vi "Meter-FunctionalTest.vi"(8 "error in (no error)":errorcluster, 11 "Meter-Test in":refnum<class "Meter-Test.lvclass">) -> (0 "error out":errorcluster, 3 "Meter-Test out":refnum<class "Meter-Test.lvclass">)   [LabVIEW 2013, in "Meter-Test.lvclass"]
uses:
  Meter-Test.lvclass
  Meter-Test.lvclass/Meter-Test.ctl
  Desktop/Meter test with feedack.llb/MGI Wait (U32).vi
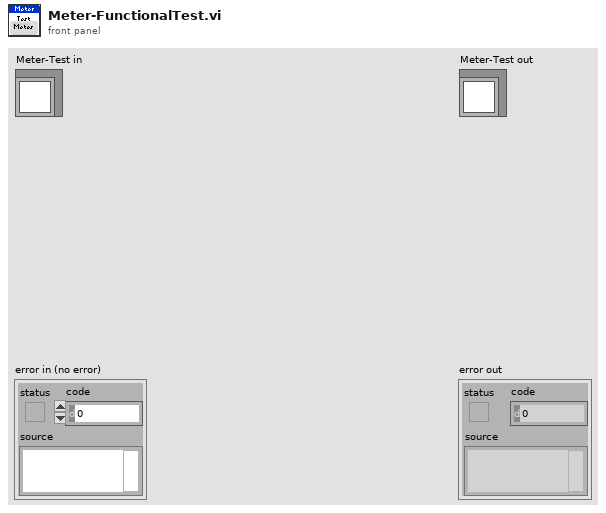
[diagram p1: front panel]
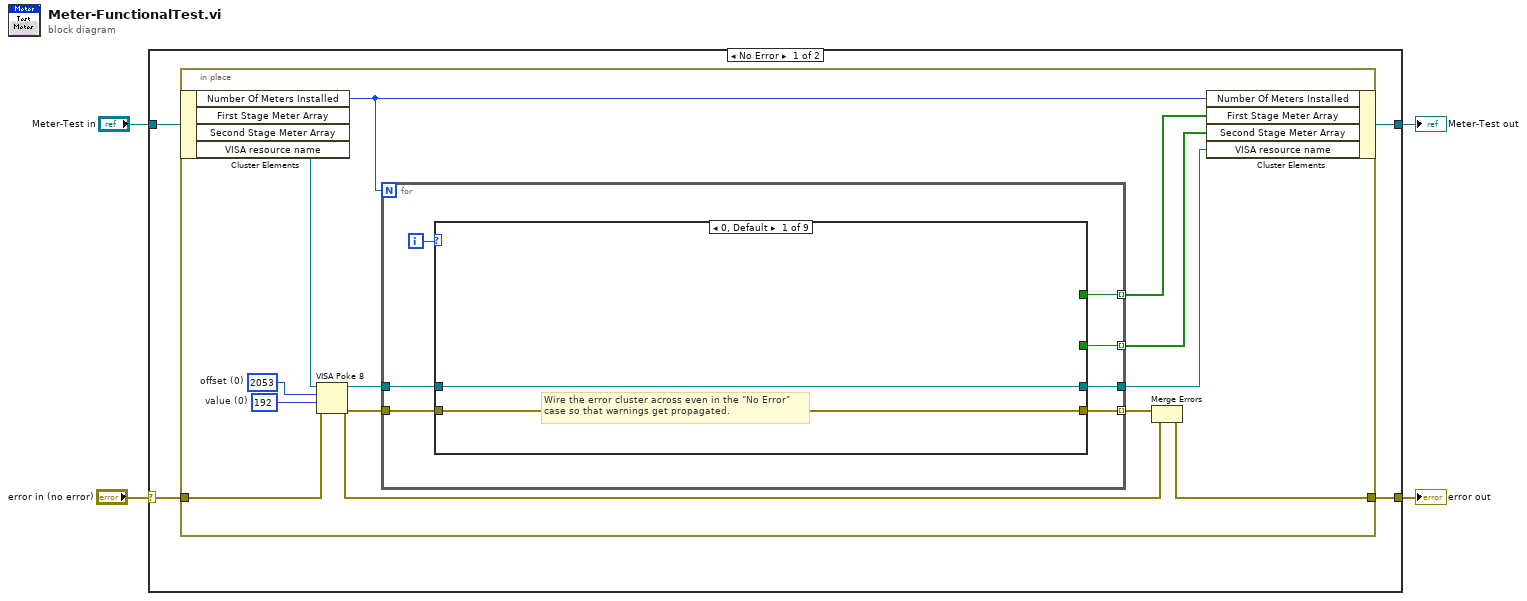
[diagram p0: block diagram]
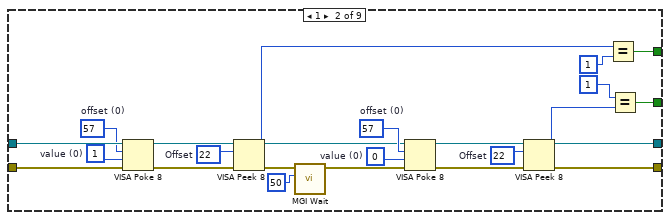
[diagram p2: hidden frame]
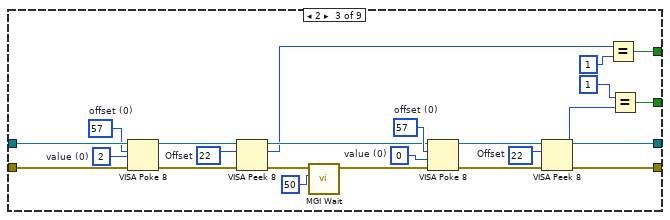
[diagram p3: hidden frame]
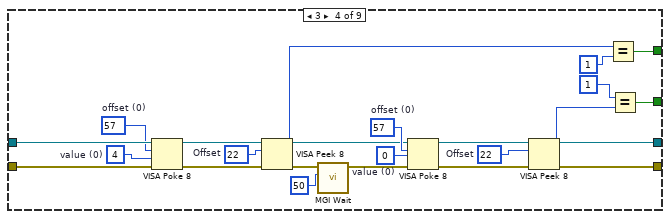
[diagram p4: hidden frame]
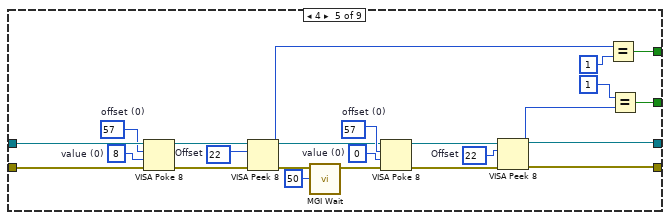
[diagram p5: hidden frame]
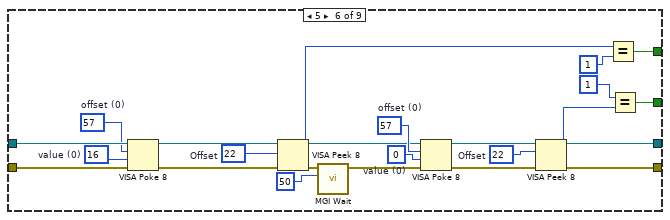
[diagram p6: hidden frame]
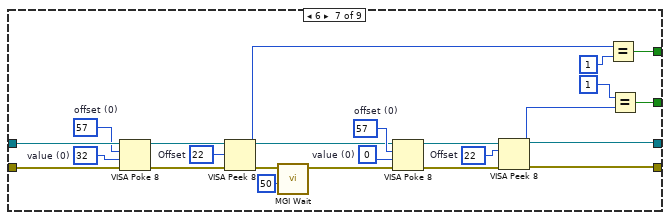
[diagram p7: hidden frame]
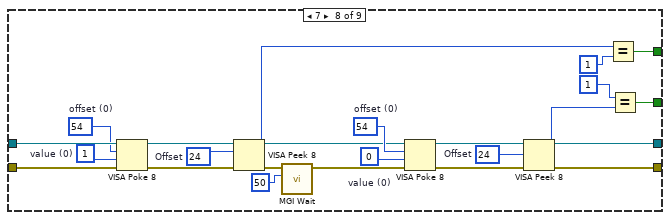
[diagram p8: hidden frame]
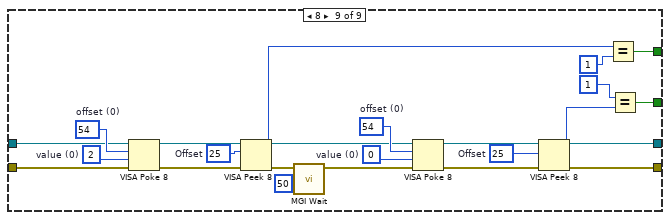
[diagram p9: hidden frame]
diagram:
  n1 = case shown="No Error" "error in (no error)" {
    selector: "error in (no error)" -> [w7 w222]
    tunnel: [w5 w222] -> w3
    tunnel: [w6 w221] -> w1
    tunnel: "Meter-Test in" -> [w8 w221]
    frame No Error {
      n2 = in-place {
        in-place-border: w7 -> [w15]
        in-place-border: [w11] -> w5
        w18 = u8 192  # value (0)
        w17 = u32 2053  # offset (0)
        # "Wire the error cluster across even in the \"No Error\"\ncase so that warnings get propagated."
        n3 = in-place-cluster #1(w8) -> ("Number Of Meters Installed"=w14:i32, "VISA resource name"=w13:refnum<visa-resource-name>)  [unwired: 2 out]
        n4 = VISA Poke 8(8:w15, 9:w18, 10:w17, 11:w13) -> (0:w20:errorcluster, 3:w16:refnum<visa-resource-name>)
        n5 = for {
          N: w14 -> [_]
          tunnel: [w27] -> w19 mode=indexing
          tunnel: w20 -> [w26]
          tunnel: w16 -> [w25]
          tunnel: [w23] -> w9 mode=indexing
          tunnel: [w22] -> w10 mode=indexing
          tunnel: [w21] -> w12
          i -> [w24]
          n6 = case shown="0, Default" w24 {
            tunnel: [w29 w52 w64 w88 w108 w132 w161 w180 w205] -> w27
            tunnel: w26 -> [w29 w51 w76 w100 w124 w148 w172 w196 w220]
            tunnel: w25 -> [w28 w50 w75 w99 w123 w147 w171 w195 w197]
            tunnel: [_ w33 w56 w80 w105 w129 w153 w177 w202] -> w23
            tunnel: [_ w30 w55 w81 w104 w128 w152 w176 w201] -> w22
            tunnel: [w28 w36 w59 w78 w101 w126 w150 w175 w200] -> w21
            frame 0, Default {
            }
            frame 1 {
              w39 = u32 22  # Offset
              w43 = u32 22  # Offset
              w45 = u8 0  # value (0)
              w46 = u32 57  # offset (0)
              w49 = u8 1  # value (0)
              w48 = u32 57  # offset (0)
              n7 = VISA Poke 8(8:w51, 9:w49, 10:w48, 11:w50) -> (0:w42:errorcluster, 3:w40:refnum<visa-resource-name>)
              n8 = VISA Peek 8(8:w42, 10:w43, 11:w40) -> (0:w41:errorcluster, 2:w31:u8, 3:w37:refnum<visa-resource-name>)
              n9 = call-poly "MGI Wait.vi"("ms"=u32 50, "Error In"=w41) -> ("Error Out"=w47:errorcluster)  [unwired: 5 in]
              n10 = VISA Poke 8(8:w47, 9:w45, 10:w46, 11:w37) -> (0:w52:errorcluster, 3:w38:refnum<visa-resource-name>)
              n11 = VISA Peek 8(10:w39, 11:w38) -> (2:w32:u8, 3:w36:refnum<visa-resource-name>)  [unwired: 1 in, 1 out]
              n12 = Equal?(x=w31, y=u8 1) -> (x = y?=w30:bool)
              n13 = Equal?(x=u8 1 ("y"), y=w32) -> (x = y?=w33:bool)
            }
            frame 2 {
              w67 = u32 22  # Offset
              w68 = u32 22  # Offset
              w70 = u8 0  # value (0)
              w71 = u32 57  # offset (0)
              w74 = u8 2  # value (0)
              w73 = u32 57  # offset (0)
              n14 = VISA Poke 8(8:w76, 9:w74, 10:w73, 11:w75) -> (0:w63:errorcluster, 3:w61:refnum<visa-resource-name>)
              n15 = VISA Peek 8(8:w63, 10:w68, 11:w61) -> (0:w62:errorcluster, 2:w54:u8, 3:w60:refnum<visa-resource-name>)
              n16 = call-poly "MGI Wait.vi"("ms"=u32 50, "Error In"=w62) -> ("Error Out"=w72:errorcluster)  [unwired: 5 in]
              n17 = VISA Poke 8(8:w72, 9:w70, 10:w71, 11:w60) -> (0:w66:errorcluster, 3:w65:refnum<visa-resource-name>)
              n18 = VISA Peek 8(8:w66, 10:w67, 11:w65) -> (0:w64:errorcluster, 2:w53:u8, 3:w59:refnum<visa-resource-name>)
              n19 = Equal?(x=w54, y=u8 1) -> (x = y?=w55:bool)
              n20 = Equal?(x=u8 1 ("y"), y=w53) -> (x = y?=w56:bool)
            }
            frame 3 {
              w92 = u32 22  # Offset
              w93 = u32 22  # Offset
              w95 = u8 0  # value (0)
              w87 = u32 57  # offset (0)
              w98 = u8 4  # value (0)
              w97 = u32 57  # offset (0)
              n21 = VISA Poke 8(8:w100, 9:w98, 10:w97, 11:w99) -> (0:w91:errorcluster, 3:w85:refnum<visa-resource-name>)
              n22 = VISA Peek 8(8:w91, 10:w93, 11:w85) -> (0:w90:errorcluster, 2:w77:u8, 3:w84:refnum<visa-resource-name>)
              n23 = call-poly "MGI Wait.vi"("ms"=u32 50, "Error In"=w90) -> ("Error Out"=w96:errorcluster)  [unwired: 5 in]
              n24 = VISA Poke 8(8:w96, 9:w95, 10:w87, 11:w84) -> (0:w89:errorcluster, 3:w86:refnum<visa-resource-name>)
              n25 = VISA Peek 8(8:w89, 10:w92, 11:w86) -> (0:w88:errorcluster, 2:w79:u8, 3:w78:refnum<visa-resource-name>)
              n26 = Equal?(x=w77, y=u8 1) -> (x = y?=w81:bool)
              n27 = Equal?(x=u8 1 ("y"), y=w79) -> (x = y?=w80:bool)
            }
            frame 4 {
              w115 = u32 22  # Offset
              w116 = u32 22  # Offset
              w118 = u8 0  # value (0)
              w119 = u32 57  # offset (0)
              w122 = u8 8  # value (0)
              w121 = u32 57  # offset (0)
              n28 = VISA Poke 8(8:w124, 9:w122, 10:w121, 11:w123) -> (0:w114:errorcluster, 3:w112:refnum<visa-resource-name>)
              n29 = VISA Peek 8(8:w114, 10:w116, 11:w112) -> (0:w113:errorcluster, 2:w103:u8, 3:w111:refnum<visa-resource-name>)
              n30 = call-poly "MGI Wait.vi"("ms"=u32 50, "Error In"=w113) -> ("Error Out"=w120:errorcluster)  [unwired: 5 in]
              n31 = VISA Poke 8(8:w120, 9:w118, 10:w119, 11:w111) -> (0:w109:errorcluster, 3:w110:refnum<visa-resource-name>)
              n32 = VISA Peek 8(8:w109, 10:w115, 11:w110) -> (0:w108:errorcluster, 2:w102:u8, 3:w101:refnum<visa-resource-name>)
              n33 = Equal?(x=w103, y=u8 1) -> (x = y?=w104:bool)
              n34 = Equal?(x=u8 1 ("y"), y=w102) -> (x = y?=w105:bool)
            }
            frame 5 {
              w139 = u32 22  # Offset
              w140 = u32 22  # Offset
              w142 = u8 0  # value (0)
              w143 = u32 57  # offset (0)
              w146 = u8 16  # value (0)
              w145 = u32 57  # offset (0)
              n35 = VISA Poke 8(8:w148, 9:w146, 10:w145, 11:w147) -> (0:w138:errorcluster, 3:w137:refnum<visa-resource-name>)
              n36 = VISA Peek 8(8:w138, 10:w140, 11:w137) -> (0:w135:errorcluster, 2:w125:u8, 3:w136:refnum<visa-resource-name>)
              n37 = call-poly "MGI Wait.vi"("ms"=u32 50, "Error In"=w135) -> ("Error Out"=w144:errorcluster)  [unwired: 5 in]
              n38 = VISA Poke 8(8:w144, 9:w142, 10:w143, 11:w136) -> (0:w133:errorcluster, 3:w134:refnum<visa-resource-name>)
              n39 = VISA Peek 8(8:w133, 10:w139, 11:w134) -> (0:w132:errorcluster, 2:w127:u8, 3:w126:refnum<visa-resource-name>)
              n40 = Equal?(x=w125, y=u8 1) -> (x = y?=w128:bool)
              n41 = Equal?(x=u8 1 ("y"), y=w127) -> (x = y?=w129:bool)
            }
            frame 6 {
              w156 = u32 22  # Offset
              w164 = u32 22  # Offset
              w166 = u8 0  # value (0)
              w167 = u32 57  # offset (0)
              w170 = u8 32  # value (0)
              w169 = u32 57  # offset (0)
              n42 = VISA Poke 8(8:w172, 9:w170, 10:w169, 11:w171) -> (0:w159:errorcluster, 3:w157:refnum<visa-resource-name>)
              n43 = VISA Peek 8(8:w159, 10:w156, 11:w157) -> (0:w160:errorcluster, 2:w149:u8, 3:w158:refnum<visa-resource-name>)
              n44 = call-poly "MGI Wait.vi"("ms"=u32 50, "Error In"=w160) -> ("Error Out"=w168:errorcluster)  [unwired: 5 in]
              n45 = VISA Poke 8(8:w168, 9:w166, 10:w167, 11:w158) -> (0:w163:errorcluster, 3:w162:refnum<visa-resource-name>)
              n46 = VISA Peek 8(8:w163, 10:w164, 11:w162) -> (0:w161:errorcluster, 2:w151:u8, 3:w150:refnum<visa-resource-name>)
              n47 = Equal?(x=w149, y=u8 1) -> (x = y?=w152:bool)
              n48 = Equal?(x=u8 1 ("y"), y=w151) -> (x = y?=w153:bool)
            }
            frame 7 {
              w188 = u32 24  # Offset
              w187 = u32 24  # Offset
              w190 = u8 0  # value (0)
              w191 = u32 54  # offset (0)
              w194 = u8 1  # value (0)
              w193 = u32 54  # offset (0)
              n49 = VISA Poke 8(8:w196, 9:w194, 10:w193, 11:w195) -> (0:w184:errorcluster, 3:w183:refnum<visa-resource-name>)
              n50 = VISA Peek 8(8:w184, 10:w188, 11:w183) -> (0:w181:errorcluster, 2:w173:u8, 3:w182:refnum<visa-resource-name>)
              n51 = call-poly "MGI Wait.vi"("ms"=u32 50, "Error In"=w181) -> ("Error Out"=w192:errorcluster)  [unwired: 5 in]
              n52 = VISA Poke 8(8:w192, 9:w190, 10:w191, 11:w182) -> (0:w186:errorcluster, 3:w185:refnum<visa-resource-name>)
              n53 = VISA Peek 8(8:w186, 10:w187, 11:w185) -> (0:w180:errorcluster, 2:w174:u8, 3:w175:refnum<visa-resource-name>)
              n54 = Equal?(x=w173, y=u8 1) -> (x = y?=w176:bool)
              n55 = Equal?(x=u8 1 ("y"), y=w174) -> (x = y?=w177:bool)
            }
            frame 8 {
              w213 = u32 25  # Offset
              w212 = u32 25  # Offset
              w215 = u8 0  # value (0)
              w216 = u32 54  # offset (0)
              w219 = u8 2  # value (0)
              w218 = u32 54  # offset (0)
              n56 = VISA Poke 8(8:w220, 9:w219, 10:w218, 11:w197) -> (0:w211:errorcluster, 3:w210:refnum<visa-resource-name>)
              n57 = VISA Peek 8(8:w211, 10:w213, 11:w210) -> (0:w208:errorcluster, 2:w198:u8, 3:w209:refnum<visa-resource-name>)
              n58 = call-poly "MGI Wait.vi"("ms"=u32 50, "Error In"=w208) -> ("Error Out"=w217:errorcluster)  [unwired: 5 in]
              n59 = VISA Poke 8(8:w217, 9:w215, 10:w216, 11:w209) -> (0:w206:errorcluster, 3:w207:refnum<visa-resource-name>)
              n60 = VISA Peek 8(8:w206, 10:w212, 11:w207) -> (0:w205:errorcluster, 2:w199:u8, 3:w200:refnum<visa-resource-name>)
              n61 = Equal?(x=w198, y=u8 1) -> (x = y?=w201:bool)
              n62 = Equal?(x=u8 1 ("y"), y=w199) -> (x = y?=w202:bool)
            }
          }
        }
        n63 = Merge Errors(w19, w20) -> (w11:errorcluster)
        n64 = in-place-cluster #1("Number Of Meters Installed"=w14, "First Stage Meter Array"=w10, "Second Stage Meter Array"=w9, "VISA resource name"=w12) -> (w6:refnum<class "Meter-Test.lvclass">)
      }
    }
    frame Error {
    }
  }
  "error out" <- w3
  "Meter-Test out" <- w1
